vi "Test_ListColumns_WorksNoError.vi"(8 "error in (no error)":errorcluster, 11 "TestCase in":refnum<class "Test mysql.lvclass">) -> (0 "error out":errorcluster, 3 "TestCase out":refnum<class "Test mysql.lvclass">)   [LabVIEW 2020, in "DataBase_mysql_Tests.lvlib" / "Test mysql.lvclass"]
uses:
  Test mysql.lvclass
  externals/mysql/Source/mysql.net/mysql.lvclass
  <vilib>/addons/_JKI Toolkits/VI Tester/TestCase.llb/TestCase.lvclass
  C:/Program Files/National Instruments/LabVIEW 2020/vi.lib/addons/_JKI Toolkits/VI Tester/TestCase.llb/TestCase.lvclass
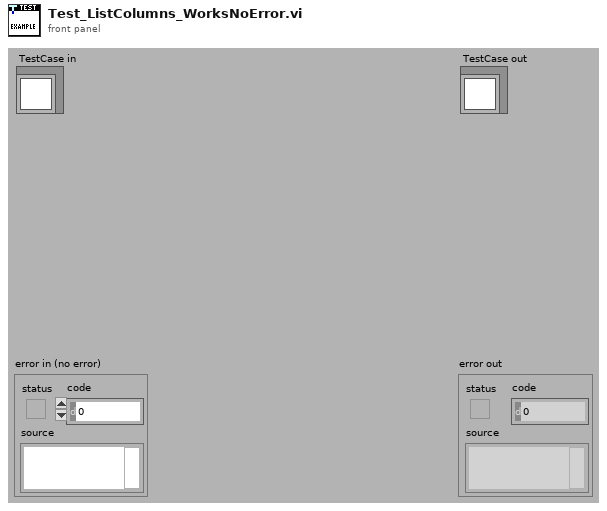
[diagram p1: front panel]
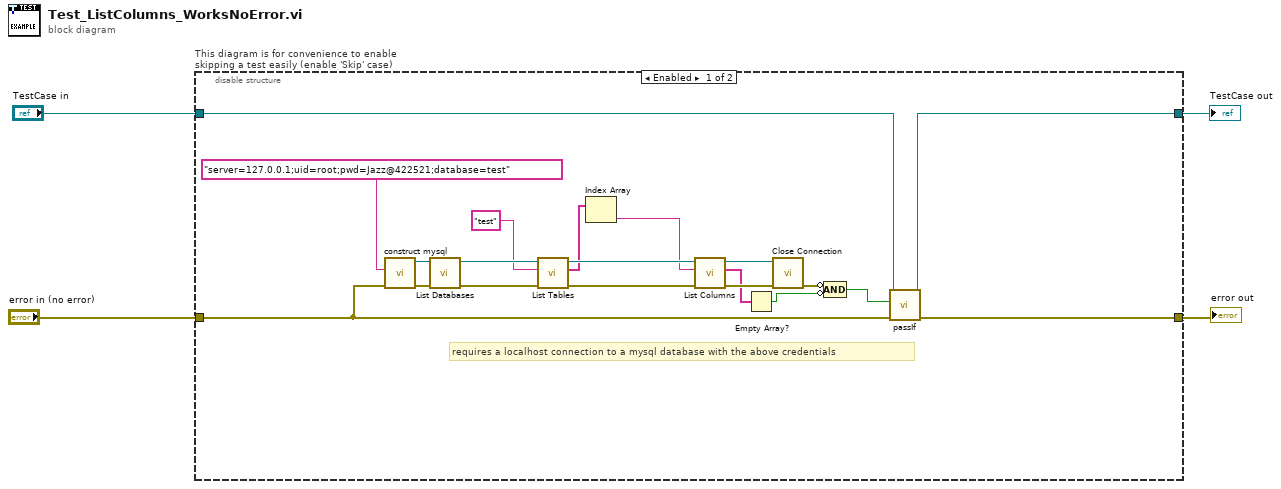
[diagram p0: block diagram]
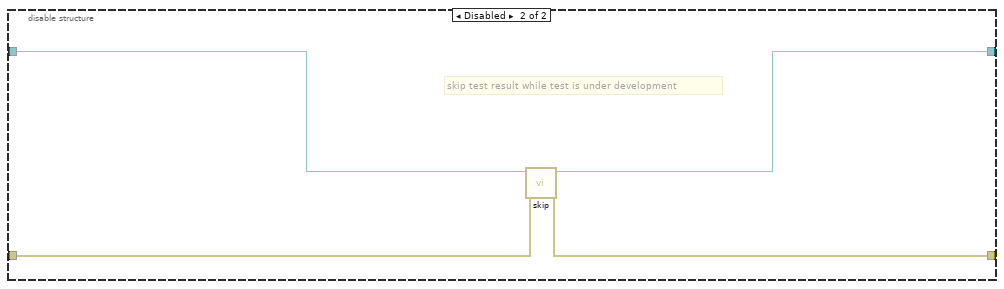
[diagram p2: hidden frame]
diagram:
  n1 = disable-structure "This diagram is for convenience to enable skipping a test easily (enable 'Skip' case)" shown="Enabled" {
    disable-tunnel: "TestCase in" -> [w24 w28]
    disable-tunnel: [w23 w26] -> w1
    disable-tunnel: [w22 w27] -> w3
    disable-tunnel: "error in (no error)" -> [w20 w25]
    frame Enabled {
      # "requires a localhost connection to a mysql database with the above credentials"
      n2 = call "construct mysql.vi"("error in (no error)"=w20, "Connection string"="server=127.0.0.1;uid=root;pwd=Jazz@422521;database=test") -> ("error out"=w16:errorcluster, "mysql out"=w15:refnum<class "mysql.lvclass">)  [unwired: 8 in]
      n3 = call-dynamic "List Databases.vi"("error in (no error)"=w16, "mysql in"=w15) -> ("error out"=w13:errorcluster, "mysql out"=w14:refnum<class "mysql.lvclass">)  [unwired: 7 in, 1 out]
      n4 = call-dynamic "List Tables.vi"("error in (no error)"=w13, "database"="test", "mysql in"=w14) -> ("error out"=w12:errorcluster, "tables"=w8:string[], "mysql out"=w10:refnum<class "mysql.lvclass">)  [unwired: 6 in]
      n5 = Index Array(array=w8) -> (element=w6:string)  [unwired: 1 in]
      n6 = call-dynamic "List Columns.vi"("error in (no error)"=w12, "schema.table in"=w6, "mysql in"=w10) -> ("error out"=w11:errorcluster, "Columns out"=w7:string[], "mysql out"=w9:refnum<class "mysql.lvclass">)  [unwired: 5 in, 1 out]
      n7 = Empty Array?(array=w7) -> (empty?=w17:bool)
      n8 = call-dynamic "Close Connection.vi"("error in (no error)"=w11, "mysql in"=w9) -> ("error out"=w19:errorcluster)  [unwired: 8 in, 1 out]
      n9 = Compound Arithmetic op=AND(invert w19, invert w17) -> (w18:bool)
      n10 = call-dynamic "passIf.vi"("error in (no error)"=w20, "pass"=w18, "TestCase in"=w24) -> ("error out"=w22:errorcluster, "TestCase out"=w23:refnum<class "Test mysql.lvclass">)  [unwired: 7 in]
    }
    frame Disabled {
      # "skip test result while test is under development"
      n11 = call <vilib>:"skip.vi"("error in (no error)"=w25, "TestCase in"=w28) -> ("error out"=w27:errorcluster, "TestCase out"=w26:refnum<class "Test mysql.lvclass">)  [unwired: 8 in]
    }
  }
  "error out" <- w3
  "TestCase out" <- w1
